vi "Capture Peak Index (Angle) (SubVI).vi"(8 "Angle":fxp<+/-,16,3> format="%.14g", 9 "Peak Index":u16, 10 "Dip Valid?":bool, 11 "Peak Count":u16) -> (3 "Peaks":T1 {"Angle" format="%.14g"})   [LabVIEW 2015]
uses:
  Controls (FPGA)/Peak Index Angle.ctl
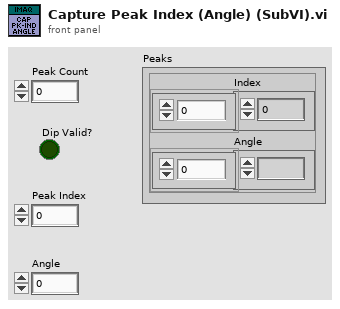
[diagram p1: front panel]
types:
  T1 = typedef "Peak Index Angle.ctl" = cluster{"Index":u16[], "Angle":fxp<+/-,16,3>[]}
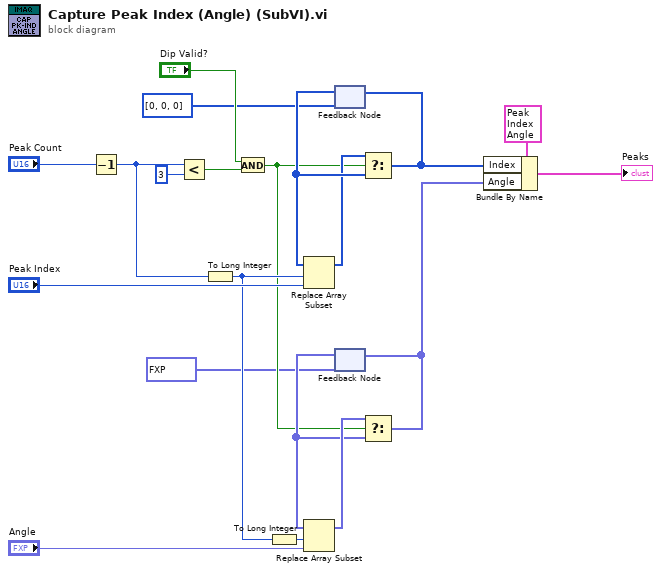
[diagram p0: block diagram]
diagram:
  n1 = Decrement(x="Peak Count") -> (x-1=w18:u16)
  n2 = Less?(x=w18, y=u16 3) -> (x < y?=w17:bool)
  n3 = To Long Integer(number=w18) -> (32bit integer=w7:i32)
  n4 = And(x="Dip Valid?", y=w17) -> (x .and. y?=w6:bool)
  n5 = To Long Integer(number=w7) -> (32bit integer=w11:i32)
  n6 = feedback #1(u16[] [0, 0, 0]) -> (w16:u16[])
  n7 = Replace Array Subset(array=w16, new element="Peak Index", index=w7) -> (w14:u16[])
  n8 = feedback #2(fxp<+/-,16,3>[] [0.0, 0.0, 0.0]) -> (w9:fxp<+/-,16,3>[])
  n9 = Replace Array Subset(array=w9, new element="Angle", index=w11) -> (w10:fxp<+/-,16,3>[])
  n10 = Select(t=w14, s=w6, f=w16) -> (s? t:f=w4:u16[])
  n11 = feedback-in #1(w4) -> ()
  n12 = Select(t=w10, s=w6, f=w9) -> (s? t:f=w2:fxp<+/-,16,3>[])
  n13 = feedback-in #2(w2) -> ()
  n14 = Bundle By Name(cluster=T1 {"Index"=[0, 0, 0], "Angle"=[0.0, 0.0, 0.0]}, "Index"=w4, "Angle"=w2) -> (→"Peaks":T1)
